vi "Fetch Full Documentation.vi"(8 "error in (no error)":errorcluster {"code" format="Error %.0f"}, 10 "File Paths":path[](array[path]), 11 "VIDoc Parser In":refnum<class "VIDoc Parser.lvclass">) -> (0 "error out":errorcluster {"code" format="Error %.0f"}, 2 "Full Documentation":T1, 3 "VIDoc Parser Out":refnum<class "VIDoc Parser.lvclass">)   [LabVIEW 2023, in "VIDoc Parsing.lvlib" / "VIDoc Parser.lvclass"]
uses:
  VIDoc Parser.lvclass
  VIDoc Parser.lvclass/VIDoc Parser.ctl
  Project Documentation/Project Documentation.lvclass
  Interface Documenation/Interface Documenation.lvclass
  Class Documentation/Class Documentation.lvclass
  Library Documentation/Library Documentation.lvclass
  GUI Documentation/GUI Documentation.lvclass
  TypeDefs/Full Documentation Info.ctl
  VIDoc Parsing.lvlib
  LLB Documentation/LLB Documentation.lvclass
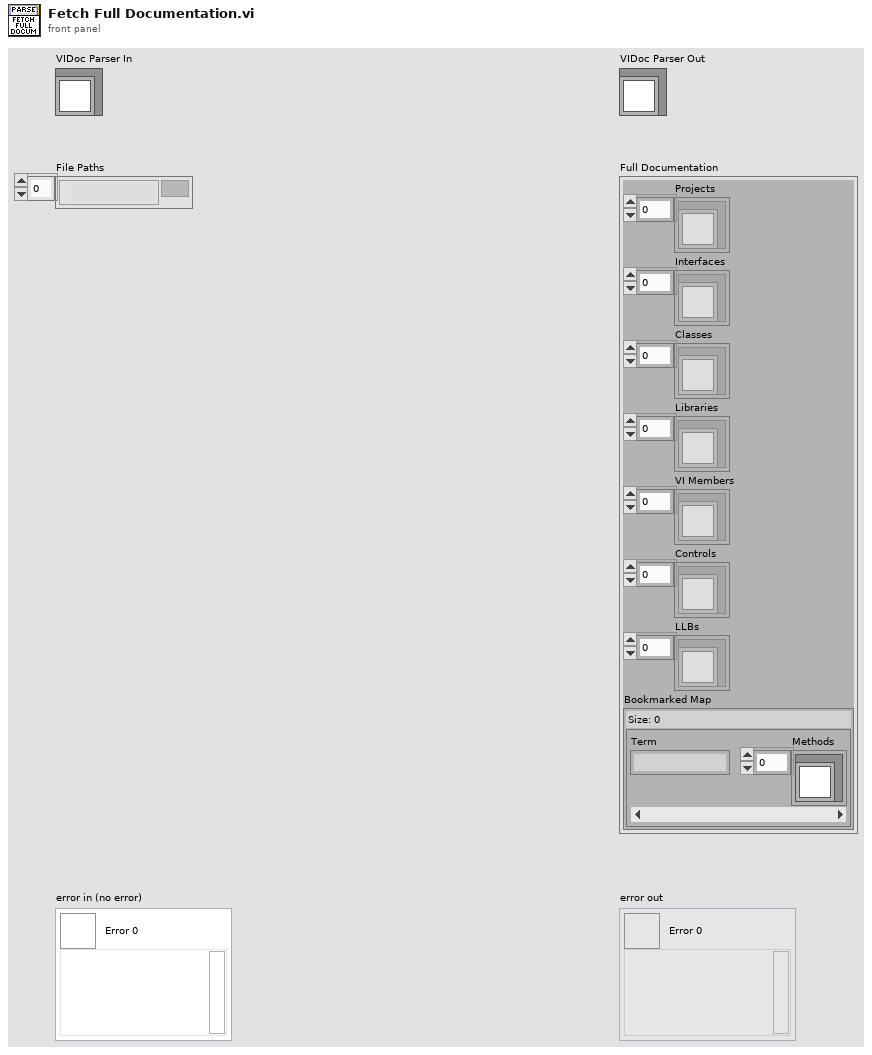
[diagram p1: front panel]
types:
  T1 = typedef "VIDoc Parsing.lvlib/Full Documentation Info.ctl" = cluster{"Projects":refnum<class "Project Documentation.lvclass">[], "Interfaces":refnum<class "Interface Documenation.lvclass">[], "Classes":refnum<class "Class Documentation.lvclass">[], "Libraries":refnum<class "Library Documentation.lvclass">[], "VI Members":refnum<class "GUI Documentation.lvclass">[], "Controls":refnum<class "GUI Documentation.lvclass">[], "LLBs":refnum<class "LLB Documentation.lvclass">[], "Bookmarked Map":map{string, refnum<class "GUI Documentation.lvclass">[]}}
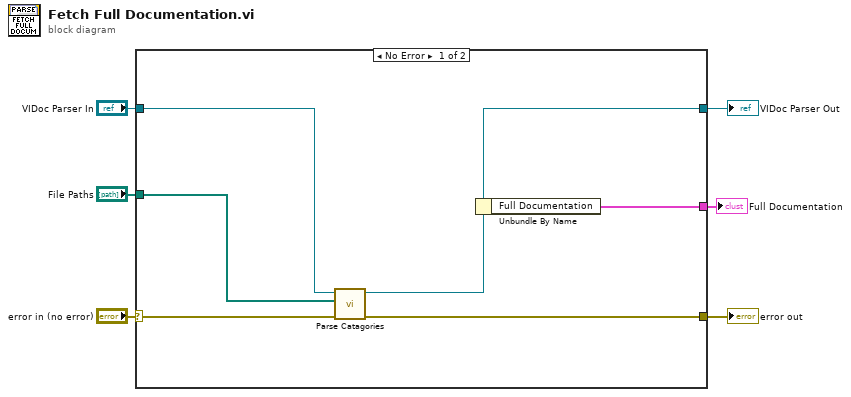
[diagram p0: block diagram]
diagram:
  n1 = case shown="No Error" "error in (no error)" {
    selector: "error in (no error)" -> [w11 w14]
    tunnel: [w9 w14] -> w5
    tunnel: [w8 w13] -> w3
    tunnel: "VIDoc Parser In" -> [w12 w13]
    tunnel: "File Paths" -> [w10 _]
    tunnel: [w7 _] -> w1
    frame No Error {
      n2 = call "Parse Catagories.vi"("error in (no error)"=w11, "File Paths"=w10, "VIDoc Parser In"=w12) -> ("error out"=w9:errorcluster, "VIDoc Parser Out"=w8:refnum<class "VIDoc Parser.lvclass">)  [unwired: 7 in]
      n3 = Unbundle By Name(w8) -> ("Full Documentation"=w7:T1)
    }
    frame Error {
    }
  }
  "error out" <- w5
  "VIDoc Parser Out" <- w3
  "Full Documentation" <- w1
